vi "GetQCPCoordinates.vi"(10 "Stop Point":T1, 11 "Start Point":T1) -> (2 "X coordinates":dbl[](array[numeric]), 3 "Y coodinates":dbl[](array[numeric]))   [LabVIEW 2017]
uses:
  KeyPoints.ctl
  <userlib>/836-Library/System/QCP_V2/QCPSupportCode/QCPData.ctl
  <userlib>/836-Library/System/QCP_V2/QCPSupportCode/QCP_GetDblArr.vi
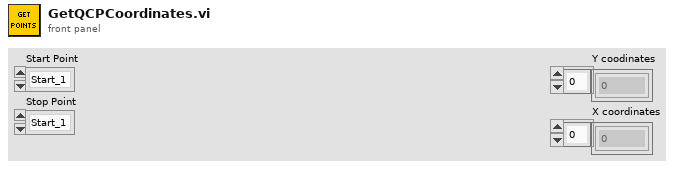
[diagram p1: front panel]
types:
  T1 = typedef "KeyPoints.ctl" = enum16{"Start_1", "Start_2", "Start_3", "Switch_L", "Switch_R", "Scale_L", "Scale_R", "Cube_1", "Cube_2", "Cube_3", "Cube_4", "Cube_5", "Cube_6", "CubeAcq_L", "CubeAcq_R", "Switch_Back_L", "Switch_Back_R"}
  T2 = typedef "Semaphore RefNum" = refnum<k1>
  T3 = cluster{"Data Value Refnum":refnum<data-value>, "semaphore":T2}
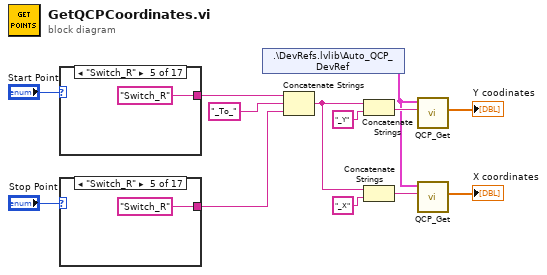
[diagram p0: block diagram]
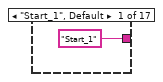
[diagram p2: hidden frame]
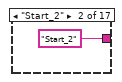
[diagram p3: hidden frame]
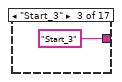
[diagram p4: hidden frame]
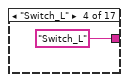
[diagram p5: hidden frame]
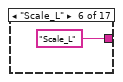
[diagram p6: hidden frame]
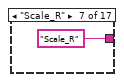
[diagram p7: hidden frame]
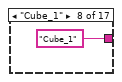
[diagram p8: hidden frame]
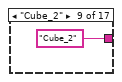
[diagram p9: hidden frame]
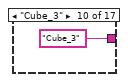
[diagram p10: hidden frame]
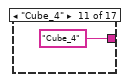
[diagram p11: hidden frame]
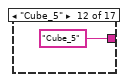
[diagram p12: hidden frame]
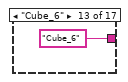
[diagram p13: hidden frame]
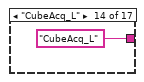
[diagram p14: hidden frame]
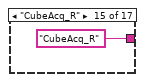
[diagram p15: hidden frame]
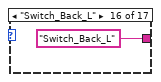
[diagram p16: hidden frame]
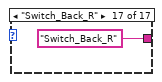
[diagram p17: hidden frame]
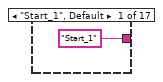
[diagram p18: hidden frame]
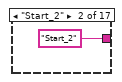
[diagram p19: hidden frame]
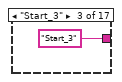
[diagram p20: hidden frame]
diagram:
  n1 = case shown="\"Switch_R\"" "Start Point" {
    tunnel: ["Start_1" "Start_2" "Start_3" "Switch_L" "Switch_R" "Scale_L" "Scale_R" "Cube_1" "Cube_2" "Cube_3" "Cube_4" "Cube_5" "Cube_6" "CubeAcq_L" "CubeAcq_R" "Switch_Back_L" "Switch_Back_R"] -> w12
    frame "Start_1", Default {
    }
    frame "Start_2" {
    }
    frame "Start_3" {
    }
    frame "Switch_L" {
    }
    frame "Switch_R" {
    }
    frame "Scale_L" {
    }
    frame "Scale_R" {
    }
    frame "Cube_1" {
    }
    frame "Cube_2" {
    }
    frame "Cube_3" {
    }
    frame "Cube_4" {
    }
    frame "Cube_5" {
    }
    frame "Cube_6" {
    }
    frame "CubeAcq_L" {
    }
    frame "CubeAcq_R" {
    }
    frame "Switch_Back_L" {
    }
    frame "Switch_Back_R" {
    }
  }
  n2 = case shown="\"Switch_R\"" "Stop Point" {
    tunnel: ["Start_1" "Start_2" "Start_3" "Switch_L" "Switch_R" "Scale_L" "Scale_R" "Cube_1" "Cube_2" "Cube_3" "Cube_4" "Cube_5" "Cube_6" "CubeAcq_L" "CubeAcq_R" "Switch_Back_L" "Switch_Back_R"] -> w9
    frame "Start_1", Default {
    }
    frame "Start_2" {
    }
    frame "Start_3" {
    }
    frame "Switch_L" {
    }
    frame "Switch_R" {
    }
    frame "Scale_L" {
    }
    frame "Scale_R" {
    }
    frame "Cube_1" {
    }
    frame "Cube_2" {
    }
    frame "Cube_3" {
    }
    frame "Cube_4" {
    }
    frame "Cube_5" {
    }
    frame "Cube_6" {
    }
    frame "CubeAcq_L" {
    }
    frame "CubeAcq_R" {
    }
    frame "Switch_Back_L" {
    }
    frame "Switch_Back_R" {
    }
  }
  n3 = shared-variable ".\\DevRefs.lvlib\\Auto_QCP_DevRef"() -> (w1:T3)  [unwired: 1 in, 1 out]
  n4 = Concatenate Strings(w12, "_To_" ("string"), w9) -> (w8:string)
  n5 = Concatenate Strings(w8, "_Y" ("string")) -> (w5:string)
  n6 = Concatenate Strings(w8, "_X" ("string")) -> (w4:string)
  n7 = call-poly <userlib>:"QCP_Get.vi"("Value Name"=w5, "QCP_DevRef_In"=w1) -> ("Values"=→"Y coodinates":dbl[])  [unwired: 7 in, 2 out]
  n8 = call-poly <userlib>:"QCP_Get.vi"("Value Name"=w4, "QCP_DevRef_In"=w1) -> ("Values"=→"X coordinates":dbl[])  [unwired: 7 in, 2 out]
